vi "openConnection.vi"(8 "error in (no error)":errorcluster, 11 "OvenController in":refnum<class "OvenController.lvclass">) -> (0 "error out":errorcluster, 3 "OvenController out":refnum<class "OvenController.lvclass">)   [LabVIEW 2023, in "AbstractFactory.lvlib" / "OvenController.lvclass"]
uses:
  OvenController.lvclass
  OvenController.lvclass/OvenController.ctl
  IConnection/IConnection.lvclass
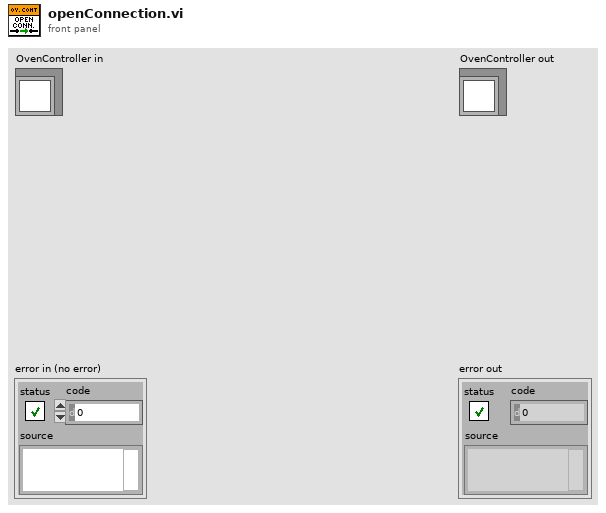
[diagram p1: front panel]
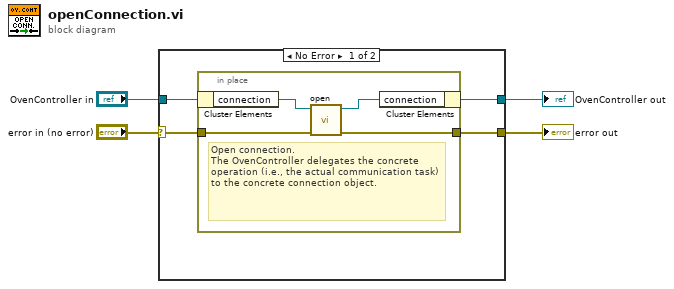
[diagram p0: block diagram]
diagram:
  n1 = case shown="No Error" "error in (no error)" {
    selector: "error in (no error)" -> [w6 w14]
    tunnel: [w5 w14] -> w3
    tunnel: [w8 w13] -> w1
    tunnel: "OvenController in" -> [w7 w13]
    frame No Error {
      n2 = in-place {
        in-place-border: w6 -> [w10]
        in-place-border: [w9] -> w5
        # "Open connection. \nThe OvenController delegates the concrete operation (i.e., the actual communication task) to the concrete connection object."
        n3 = in-place-cluster #1(w7) -> ("connection"=w12:refnum<class "IConnection.lvclass">)
        n4 = call-dynamic "open.vi"("error in (no error)"=w10, "IConnection in"=w12) -> ("error out"=w9:errorcluster, "IConnection out"=w11:refnum<class "IConnection.lvclass">)  [unwired: 8 in]
        n5 = in-place-cluster #1("connection"=w11) -> (w8:refnum<class "OvenController.lvclass">)
      }
    }
    frame Error {
    }
  }
  "error out" <- w3
  "OvenController out" <- w1
